vi "SCD - Trigger Sequence - Calculate 2kHz Waveform.vi"(8 "error in":errorcluster, 10 "Total Time (ms)":dbl=200.0, 11 "Voltages":dbl[](array[numeric])=[0.5, 1.0, 1.5, 2.0, 2.5] format="%.3g") -> (0 "error out":errorcluster, 3 "tuning waveforms":waveform(dbl)[](array[waveform])=[{"t0"=timestamp(0 s since 1904-01-01), "dt"=0.000125, "Y"=array[1600 elements]}, {"t0"=timestamp(0 s since 1904-01-01), "dt"=0.000125, "Y"=array[1600 elements]}, {"t0"=timestamp(0 s since 1904-01-01), "dt"=0.000125, "Y"=array[1600 elements]}, {"t0"=timestamp(0 s since 1904-01-01), "dt"=0.000125, "Y"=array[1600 elements]}, {"t0"=timestamp(0 s since 1904-01-01), "dt"=0.000125, "Y"=array[1600 elements]}])   [LabVIEW 2014]
doc: "This VI generates the analog waveforms necessary to tune the Lyot filter to a particular wavelength. The wavelength is controlled by the 2kHz AC (0-10 Vrms) analog voltages applied to each of 4 nematic liquid crystals from Meadowlark Optics.\n\nThe sampling information for this VI is generated externally in the calling VI which generates the polarization modulation waveforms applied to the FLC liquid crystals."
uses:
  <vilib>/measure/NI_MABase.lvlib
panel:
  out "Waveform Graph":waveform(dbl)[](graph)=[{"t0"=timestamp(0 s since 1904-01-01), "dt"=0.000125, "Y"=array[1600 elements]}, {"t0"=timestamp(0 s since 1904-01-01), "dt"=0.000125, "Y"=array[1600 elements]}, {"t0"=timestamp(0 s since 1904-01-01), "dt"=0.000125, "Y"=array[1600 elements]}, {"t0"=timestamp(0 s since 1904-01-01), "dt"=0.000125, "Y"=array[1600 elements]}, {"t0"=timestamp(0 s since 1904-01-01), "dt"=0.000125, "Y"=array[1600 elements]}]
  # "This VI is almost identical to that for PDSS.  It differs only in that SCD\nhas 5 nematic Liquid Crystals in it's Lyot Filter whereas PDSS/CoMP-S has 4\nematic LC's require a modulation frequency of 2 kHz.  \n\nFor a 2kHz waveform defined by 4 points per cycle, \nwe need a 8000 AO points per second sampling Frequency (Fs).  This means the hardsware\nupdates DAQ voltages every 125 microseconds.   \n\nA single LCVR modulation cycle (4 points) requires 500 microseconds.\n\nA 0.2 seconds modulation requires 1600 point (0.2 / 0.000125)\n\nMatus and Scott selected 0.2 seconds because this is equal to the relaxation time\nof the LCVR's and creates a nice 'brick' for constructing long series of voltages"
  # "Liquid Crystal Variable Retarders"
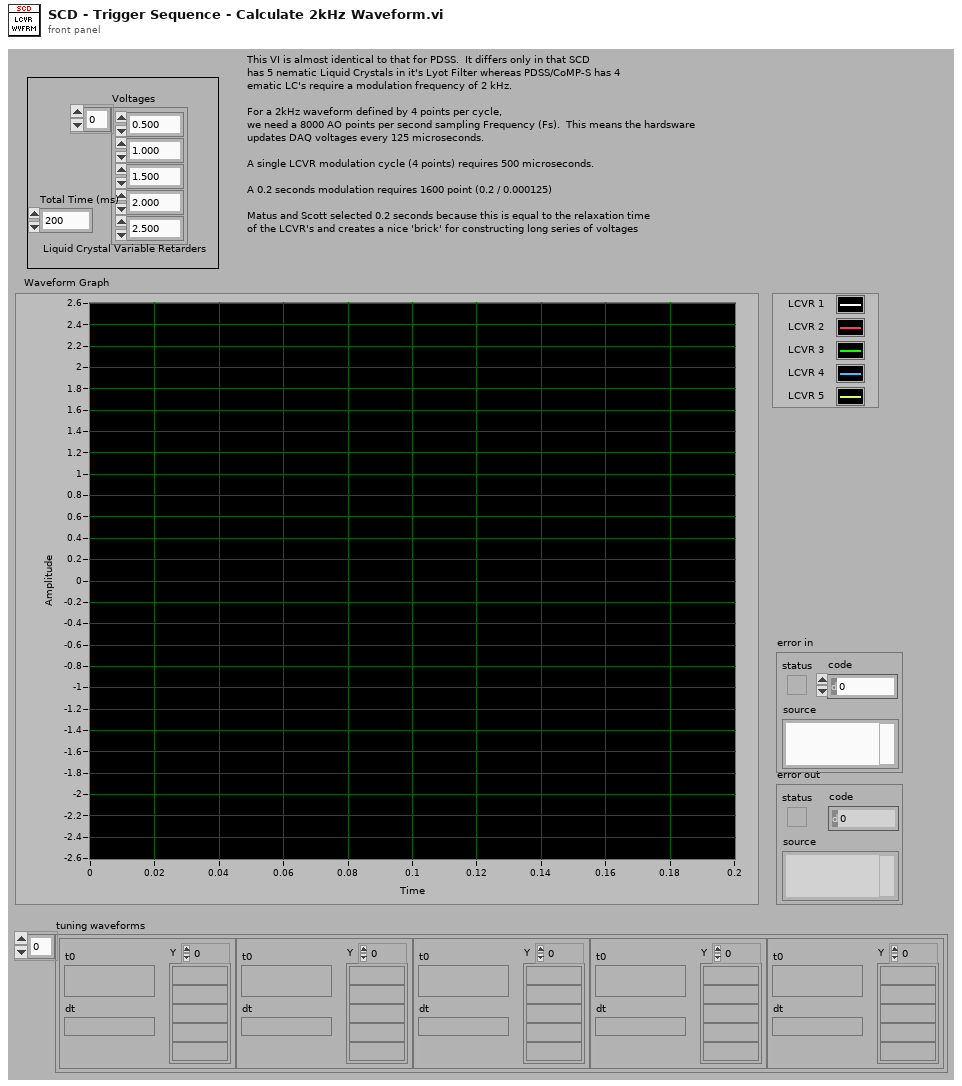
[diagram p1: front panel]
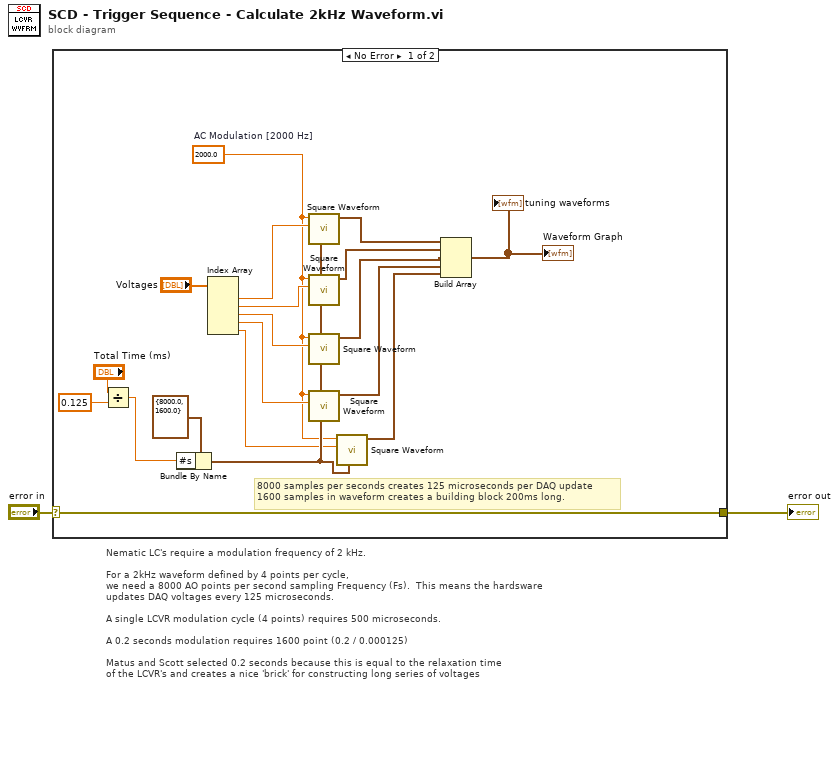
[diagram p0: block diagram]
diagram:
  # "Nematic LC's require a modulation frequency of 2 kHz.  \n\nFor a 2kHz waveform defined by 4 points per cycle, \nwe need a 8000 AO points per second sampling Frequency (Fs).  This means the hardsware\nupdates DAQ voltages every 125 microseconds.   \n\nA single LCVR modulation cycle (4 points) requires 500 microseconds.\n\nA 0.2 seconds modulation requires 1600 point (0.2 / 0.000125)\n\nMatus and Scott selected 0.2 seconds because this is equal to the relaxation time\nof the LCVR's and creates a nice 'brick' for constructing long series of voltages"
  n1 = case shown="No Error" "error in" {
    selector: "error in" -> [w21 w22]
    tunnel: [w21 w22] -> w1
    frame No Error {
      w4 = 2000.0  # AC Modulation [2000 Hz]
      # "8000 samples per seconds creates 125 microseconds per DAQ update\n1600 samples in waveform creates a building block 200ms long."
      n2 = Divide(x="Total Time (ms)", y=0.125) -> (x/y=w7:dbl)
      n3 = Bundle By Name(cluster=cluster{"Fs":dbl, "#s":dbl} {"Fs"=8000.0, "#s"=1600.0} ("sampling info"), "#s"=w7) -> (w6:cluster{"Fs":dbl, "#s":dbl})
      n4 = Index Array(array="Voltages") -> (element #1=w14:dbl, element #2=w13:dbl, element #3=w12:dbl, element #4=w11:dbl, element #5=w5:dbl)  [unwired: 5 in]
      n5 = call <vilib>:"Square Waveform.vi"("sampling info"=w6, "amplitude"=w14, "frequency"=w4) -> ("signal out"=w19:waveform(dbl))  [unwired: 7 in, 1 out]
      n6 = call <vilib>:"Square Waveform.vi"("sampling info"=w6, "amplitude"=w13, "frequency"=w4) -> ("signal out"=w18:waveform(dbl))  [unwired: 7 in, 1 out]
      n7 = call <vilib>:"Square Waveform.vi"("sampling info"=w6, "amplitude"=w12, "frequency"=w4) -> ("signal out"=w17:waveform(dbl))  [unwired: 7 in, 1 out]
      n8 = call <vilib>:"Square Waveform.vi"("sampling info"=w6, "amplitude"=w11, "frequency"=w4) -> ("signal out"=w16:waveform(dbl))  [unwired: 7 in, 1 out]
      n9 = call <vilib>:"Square Waveform.vi"("sampling info"=w6, "amplitude"=w5, "frequency"=w4) -> ("signal out"=w3:waveform(dbl))  [unwired: 7 in, 1 out]
      n10 = Build Array(w19, w18, w17, w16, w3) -> (→"Waveform Graph" →"tuning waveforms":waveform(dbl)[])
    }
    frame Error {
    }
  }
  "error out" <- w1
